vi "Test Beep Actor Events.vi"() -> ()   [LabVIEW 2016, in "CS++BeepActor.lvlib"]
doc: "Test Beep Actor"
uses:
  CS++BeepActor.lvlib
  Beep.lvclass
  C:/User/Brand/LVP/TASCA/UTCS/Packages/CSPP_Core/Actors/CS++BaseActor/CS++BaseActor.lvclass
  C:/Program Files (x86)/National Instruments/LabVIEW 2016/vi.lib/ActorFramework/Actor/Actor.lvclass
  CSPP_Core/Actors/CS++BaseActor/CS++BaseActor.lvclass/CS++BaseActor.ctl
  <vilib>/ActorFramework/Message Enqueuer/Message Enqueuer.lvclass/Message Enqueuer.ctl
  Beep Messages/Write Beep Parameters Msg/Write Beep Parameters Msg.lvclass/Write Beep Parameters Msg.ctl
  CSPP_Core/Actors/CS++BaseActor Messages/Polling Start Stop Msg/Polling Start Stop Msg.lvclass/Polling Start Stop Msg.ctl
  CSPP_Core/Actors/CS++BaseActor Messages/Write Polling Iterations Msg/Polling Iterations Msg.lvclass/Polling Iterations Msg.ctl
  CSPP_Core/Actors/CS++BaseActor Messages/Polling Interval Msg/Polling Interval Msg.lvclass/Polling Interval Msg.ctl
  <vilib>/ActorFramework/Message Enqueuer/Enqueue.vi
  Beep Messages/Beep Msg/Beep Msg.lvclass
  C:/Program Files (x86)/National Instruments/LabVIEW 2016/vi.lib/ActorFramework/Message/Message.lvclass
  Beep Messages/Write Beep Parameters Msg/Write Beep Parameters Msg.lvclass
  CSPP_Core/Actors/CS++BaseActor Messages/Polling Start Stop Msg/Polling Start Stop Msg.lvclass
  CSPP_Core/Actors/CS++BaseActor Messages/Write Polling Iterations Msg/Polling Iterations Msg.lvclass
  CSPP_Core/Actors/CS++BaseActor Messages/Polling Interval Msg/Polling Interval Msg.lvclass
  <vilib>/ActorFramework/Stop Msg/Stop Msg.lvclass
  <vilib>/ActorFramework/Message Priority Queue/Priority Enqueue.vi
  CSPP_Core/Actors/CS++BaseActor/CS++BaseActor.lvclass
  <vilib>/ActorFramework/Actor/Actor.lvclass
panel:
  in  "Play Button":bool
  in  "Beep":bool
  in  "Stop":bool
  in  "Polling Iterations":u32
  in  "Polling Interval":dbl[unit]=1.0
  in  "Duration":dbl[unit]=0.1
  in  "Frequency (440)":dbl[unit]=440.0
  in  "Use System Alert?":bool
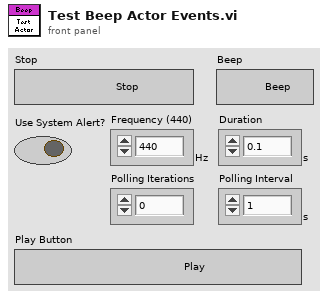
[diagram p1: front panel]
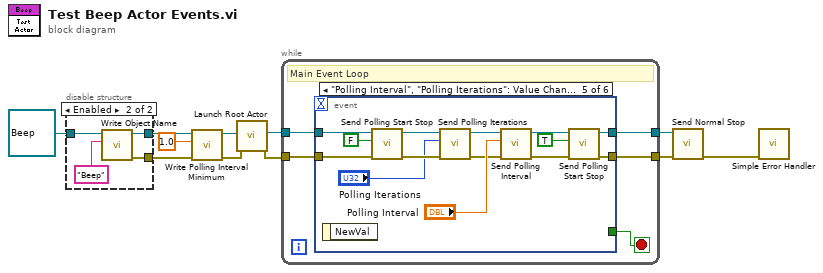
[diagram p0: block diagram]
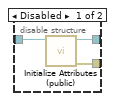
[diagram p2: hidden frame]
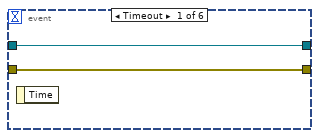
[diagram p3: hidden frame]
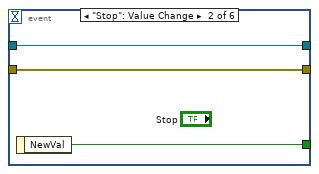
[diagram p4: hidden frame]
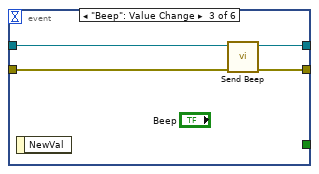
[diagram p5: hidden frame]
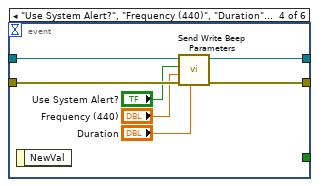
[diagram p6: hidden frame]
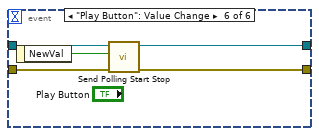
[diagram p7: hidden frame]
diagram:
  n1 = disable-structure shown="Enabled" {
    disable-tunnel: refnum<class "Beep.lvclass"> refnum ("CS++BeepActor.lvlib:Beep.lvclass") -> [w14 w18]
    disable-tunnel: [w13 w17] -> w7
    disable-tunnel: [w12 w15] -> w5
    frame Disabled {
      n2 = call "Initialize Attributes (public).vi"("CS++BaseActor in"=w14) -> ("error out"=w12:errorcluster, "CS++BaseActor out"=w13:refnum<class "Beep.lvclass">)  [unwired: 8 in, 1 out]
    }
    frame Enabled {
      n3 = call "Write Object Name.vi"("Object Name"="Beep", "CS++BaseActor in"=w18) -> ("error out"=w15:errorcluster, "CS++BaseActor out"=w17:refnum<class "Beep.lvclass">)  [unwired: 8 in]
    }
  }
  n4 = call "Write Polling Interval Minimum.vi"("error in (no error)"=w5, "Polling Interval Minimum"=dbl[unit] 1.0, "CS++BaseActor in"=w7) -> ("error out"=w3:errorcluster, "CS++BaseActor out"=w4:refnum<class "Beep.lvclass">)  [unwired: 7 in]
  n5 = call <vilib>:"Launch Root Actor.vi"("error in (no error)"=w3, "Actor"=w4) -> ("error out"=w1:errorcluster, "Actor's Enqueuer"=w2:refnum<class "Message Enqueuer.lvclass">)  [unwired: 8 in]
  n6 = while {
    tunnel: w1 -> [w20]
    tunnel: [w22] -> w11
    tunnel: w2 -> [w23]
    tunnel: [w21] -> w10
    stop <- w19 stop-if-true
    # "Main Event Loop"
    n7 = event shown="[4] \"Polling Interval\", \"Polling Iterations\": Value Change" {
      selector: _ -> [_ _ _ _ _ _]
      dyn-events: _ -> [_ _ _ _ _ _]
      timeout: _ -> [_ _ _ _ _ _]
      tunnel: w23 -> [w25 w26 w32 w39 w51 w55]
      tunnel: [w25 w26 w29 w36 w49 w58] -> w22
      tunnel: [w24 w27 w30 w37 w50 w57] -> w21
      tunnel: w20 -> [w24 w27 w31 w38 w52 w56]
      tunnel: [_ w28 _ _ _ _] -> w19
      event Timeout {
        n8 = event-data() -> ()  [unwired: 1 in, 1 out]
      }
      event "Stop": Value Change {
        n9 = event-data() -> ("NewVal"=w28:bool)  [unwired: 1 in]
      }
      event "Beep": Value Change {
        n10 = event-data() -> ()  [unwired: 1 in, 1 out]
        n11 = call "Send Beep.vi"("error in (no error)"=w31, "Message Enqueuer"=w32) -> ("error out"=w30:errorcluster, "Message Enqueuer out"=w29:refnum<class "Message Enqueuer.lvclass">)  [unwired: 8 in]
      }
      event "Use System Alert?", "Frequency (440)", "Duration": Value Change {
        n12 = event-data() -> ()  [unwired: 1 in, 1 out]
        n13 = call "Send Write Beep Parameters.vi"("Duration"="Duration", "error in (no error)"=w38, "Frequency (440)"="Frequency (440)", "Use System Alert?"="Use System Alert?", "Message Enqueuer"=w39) -> ("error out"=w37:errorcluster, "Message Enqueuer out"=w36:refnum<class "Message Enqueuer.lvclass">)  [unwired: 5 in]
      }
      event "Polling Interval", "Polling Iterations": Value Change {
        n14 = event-data() -> ()  [unwired: 1 in, 1 out]
        n15 = call "Send Polling Start Stop.vi"("error in (no error)"=w52, "Start Polling"=FALSE ("Start (F)"), "Message Enqueuer"=w51) -> ("error out"=w43:errorcluster, "Message Enqueuer out"=w44:refnum<class "Message Enqueuer.lvclass">)  [unwired: 7 in]
        n16 = call "Send Polling Iterations.vi"("error in (no error)"=w43, "Polling Iterations"="Polling Iterations", "Message Enqueuer"=w44) -> ("error out"=w42:errorcluster, "Message Enqueuer out"=w41:refnum<class "Message Enqueuer.lvclass">)  [unwired: 7 in]
        n17 = call "Send Polling Interval.vi"("error in (no error)"=w42, "Polling Interval"="Polling Interval", "Message Enqueuer"=w41) -> ("error out"=w45:errorcluster, "Message Enqueuer out"=w46:refnum<class "Message Enqueuer.lvclass">)  [unwired: 7 in]
        n18 = call "Send Polling Start Stop.vi"("error in (no error)"=w45, "Start Polling"=TRUE ("Start (F)"), "Message Enqueuer"=w46) -> ("error out"=w50:errorcluster, "Message Enqueuer out"=w49:refnum<class "Message Enqueuer.lvclass">)  [unwired: 7 in]
      }
      event "Play Button": Value Change {
        n19 = event-data() -> ("NewVal"=w54:bool)  [unwired: 1 in]
        n20 = call "Send Polling Start Stop.vi"("error in (no error)"=w56, "Start Polling"=w54, "Message Enqueuer"=w55) -> ("error out"=w57:errorcluster, "Message Enqueuer out"=w58:refnum<class "Message Enqueuer.lvclass">)  [unwired: 7 in]
      }
    }
  }
  n21 = call <vilib>:"Send Normal Stop.vi"("error in (no error)"=w10, "Message Enqueuer"=w11) -> ("error out"=w9:errorcluster)  [unwired: 9 in]
  n22 = call <vilib>:"Simple Error Handler.vi"("error in (no error)"=w9) -> ()  [unwired: 4 in, 5 out]
